vi "niFpgaLrmPalette_MergeVI_Handshake.vi"   [LabVIEW 2017]
doc: "Represents a VI-defined handshake item. Right-click the node and select <B>Configure</B> to configure the VI-defined handshake item. Use VI-defined handshake items to create reentrant subVIs and avoid resource conflicts."
uses:
  <vilib>/rvi/DataTransferAndStorage/Container/Common/niFpgaContainerGetUniqueNameForEmu.vi
  <vilib>/rvi/DataTransferAndStorage/Container/Common/niFpgaContainerSetEmuInfo.vi
  <vilib>/rvi/eio/common/nirviEmuReportErrorAndStop.vi
  <vilib>/rvi/LocalResourceManager/LocalResourceManager.xnode
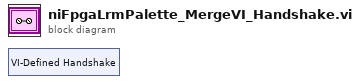
[diagram p0: block diagram]
diagram:
  n1 = xnode "VI-Defined Handshake"() -> ()  [unwired: 1 out]
